vi "SRVGlobals.vi"() -> ()   [LabVIEW 2014]
panel:
  in  "Connected SRV ID":refnum<k5>[](array[refnum])
  in  "Connected SRV IP":string[](array[string])
  in  "Buffer size (# bytes)":i32=2046
  in  "Communication":string
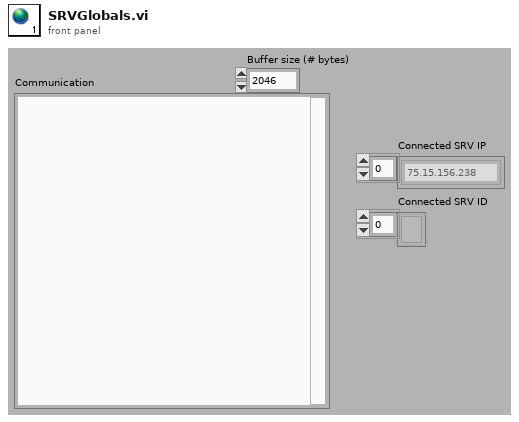
[diagram p1: front panel]
diagram:
